vi "题目1.vi"   [LabVIEW 2017]
types:
  T1 = enum16{"open", "replace", "create", "open or create", "replace or create", "replace or create with confirmation"}
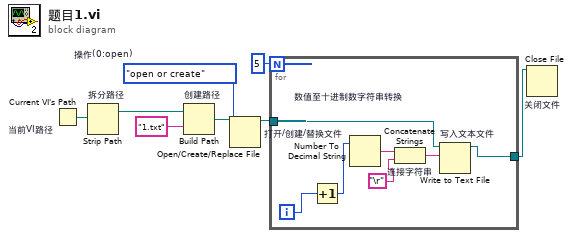
[diagram p0: block diagram]
diagram:
  w4 = T1."open or create"  # 操作(0:open)
  n1 = Current VI's Path "当前VI路径"() -> (path=w8:path)
  n2 = Strip Path "拆分路径"(path=w8) -> (stripped path=w7:path)  [unwired: 1 out]
  n3 = Build Path "创建路径"(base path=w7, name or relative path="1.txt" ("名称或相对路径")) -> (appended path=w5:path)
  n4 = Open/Create/Replace File "打开/创建/替换文件"(file path (use dialog)=w5, operation (0:open)=w4) -> (refnum out=w2:refnum<file>)  [unwired: 4 in, 2 out]
  n5 = for {
    N: 5 -> [_]
    tunnel: w2 -> [w11]
    tunnel: [w9] -> w1
    i -> [w15]
    n6 = Increment(x=w15) -> (x+1=w10:i32)
    n7 = Number To Decimal String "数值至十进制数字符串转换"(number=w10) -> (decimal integer string=w14:string)  [unwired: 1 in]
    n8 = Concatenate Strings "连接字符串"(w14, "\r") -> (w12:string)
    n9 = Write to Text File "写入文本文件"(file (use dialog)=w11, text=w12) -> (refnum out=w9:refnum<file>)  [unwired: 2 in, 2 out]
  }
  n10 = Close File "关闭文件"(refnum=w1) -> ()  [unwired: 1 in, 2 out]
